vi "Utility_Get Control Labels.vi"() -> ()   [LabVIEW 2020]
panel:
  out "spreadsheet string":string
  out "Labels":string[](array[string])
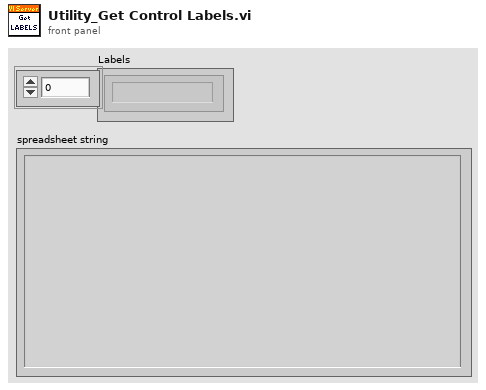
[diagram p1: front panel]
types:
  T1 = typedef "VI Server_RefsCluster.ctl" = cluster{"Labels":string[], "Refs":refnum<vi>[], "VI Ref":refnum<vi>}
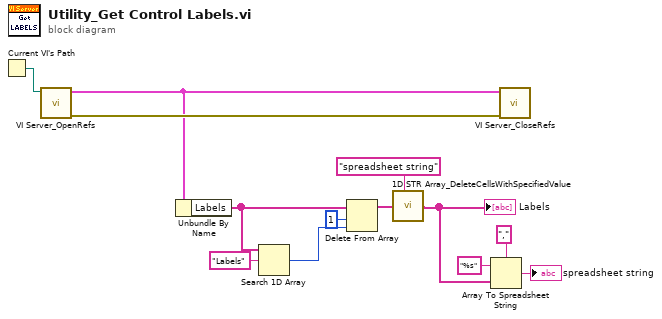
[diagram p0: block diagram]
diagram:
  n1 = Current VI's Path() -> (path=w13:path)
  n2 = call "VI Server_OpenRefs.vi"("VI Path"=w13) -> ("error out"=w12:errorcluster, "VI Server.RefsCluster"=w11:T1)  [unwired: 9 in]
  n3 = Unbundle By Name(w11) -> ("Labels"=w9:string[])
  n4 = Search 1D Array(1D array=w9, element="Labels") -> (index of element=w8:i32)  [unwired: 1 in]
  n5 = Delete From Array(array=w9, length=1, index=w8) -> (array with subset deleted=w3:string[])  [unwired: 1 out]
  n6 = call "1D STR Array_DeleteCellsWithSpecifiedValue.vi"("CellValueToBeDeleted"="spreadsheet string", "1D STR Array.IN"=w3) -> ("1D STR Array.OUT"=w1:string[])  [unwired: 5 in]
  "Labels" <- w1
  n7 = Array To Spreadsheet String(delimiter (Tab)=",", array=w1, 3:"%s" ("format string")) -> (spreadsheet string=→"spreadsheet string":string)
  n8 = call "VI Server_CloseRefs.vi"("error in"=w12, "VI Server.RefsCluster"=w11) -> ()  [unwired: 9 in, 1 out]
